vi "Write Theme.vi"(8 "error in (no error)":errorcluster, 10 "Theme.lvclass":refnum<class "Theme.lvclass">, 11 "Popup in":refnum<class "Popup.lvclass">) -> (0 "error out":errorcluster, 3 "Popup out":refnum<class "Popup.lvclass">)   [LabVIEW 2021, in "Pop-Up.lvlib" / "Popup.lvclass"]
doc: "Write the theme class for the pop up\n\n<b>Code Developed By:</b> +\nDaniel Coons +\nhttps://github.com/danielcoons/tsc-pop-up"
uses:
  Popup.lvclass
  Theme/Theme.lvclass
  Popup.lvclass/Popup.ctl
  PopUp Theme Global.vi
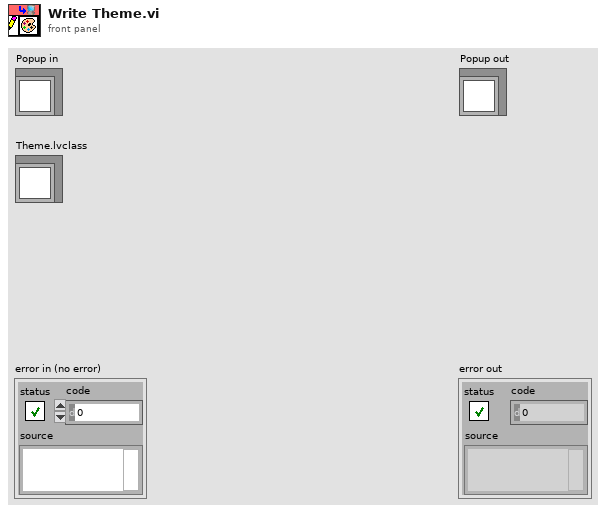
[diagram p1: front panel]
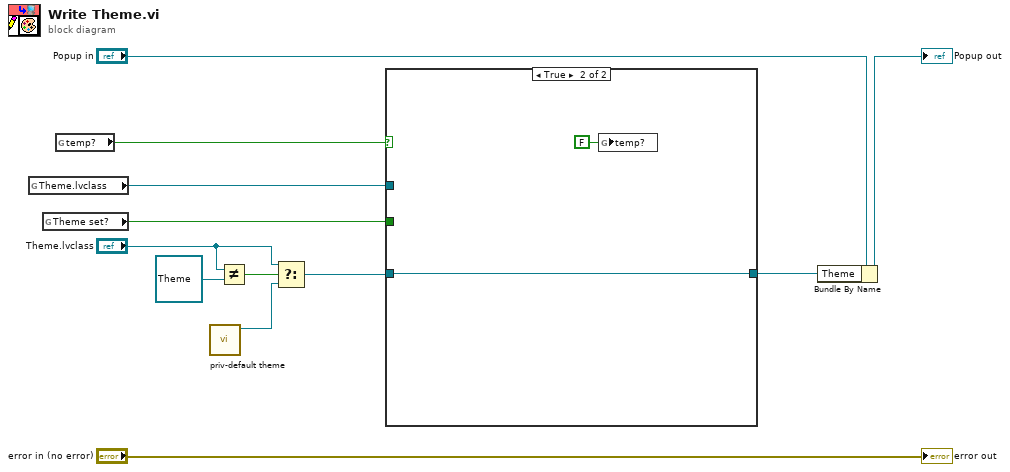
[diagram p0: block diagram]
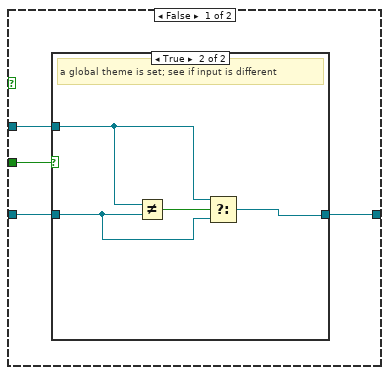
[diagram p2: hidden frame]
diagram:
  n1 = global read "PopUp Theme Global.vi" "Theme.lvclass"() -> (w8:refnum<class "Theme.lvclass">)
  n2 = global read "PopUp Theme Global.vi" "Theme set?"() -> (w9:bool)
  n3 = global read "PopUp Theme Global.vi" "temp?"() -> (w1:bool)
  n4 = call "priv-default theme.vi"() -> ("Theme out"=w5:refnum<class "Theme.lvclass">)  [unwired: 11 in]
  n5 = Not Equal?(x="Theme.lvclass", y=refnum<class "Theme.lvclass"> refnum ("Theme.lvclass")) -> (x != y?=w6:bool)
  n6 = Select(t="Theme.lvclass", s=w6, f=w5) -> (s? t:f=w3:refnum<class "Theme.lvclass">)
  n7 = case shown="True" w1 {
    tunnel: w9 -> [w16 _]
    tunnel: w8 -> [w15 _]
    tunnel: w3 -> [w14 w23]
    tunnel: [w13 w23] -> w2
    frame False {
      n8 = case shown="True" w16 {
        tunnel: w15 -> [_ w20]
        tunnel: [w17 w19] -> w13
        tunnel: w14 -> [w17 w18]
        frame False {
          # "no theme has been set"
        }
        frame True {
          # "a global theme is set; see if input is different"
          n9 = Not Equal?(x=w20, y=w18) -> (x != y?=w21:bool)
          n10 = Select(t=w20, s=w21, f=w18) -> (s? t:f=w19:refnum<class "Theme.lvclass">)
        }
      }
    }
    frame True {
      n11 = global write "PopUp Theme Global.vi" "temp?"(FALSE ("temp?")) -> ()
    }
  }
  n12 = Bundle By Name(cluster="Popup in", "Theme"=w2) -> (→"Popup out":refnum<class "Popup.lvclass">)
  "error out" <- "error in (no error)"
